vi "Init_Instr.vi"(8 "error in (no error)":errorcluster caption="entrée d'erreur (pas d'erreur)", 11 "Class Instrument Multimeter en entrée":refnum<class "Class Instrument Spectrum_Analyser.lvclass">) -> (0 "error out":errorcluster caption="sortie d'erreur", 3 "Class Instrument Multimeter en sortie":refnum<class "Class Instrument Spectrum_Analyser.lvclass">)   [LabVIEW 2020, in "Library Instrument & Equipement.lvlib" / "Library Instruments.lvlib" / "Class Instrument Spectrum_Analyser.lvclass"]
uses:
  Class Instrument Spectrum_Analyser.lvclass
  Class Instrument Spectrum_Analyser.lvclass/Class Instrument Spectrum_Analyser.ctl
  Instrument (Default)/Class Instrument (Default).lvclass
  Spectrum Analyser/Class Spectrum Analyser (Default)/Class Spectrum Analyser (Default).lvclass
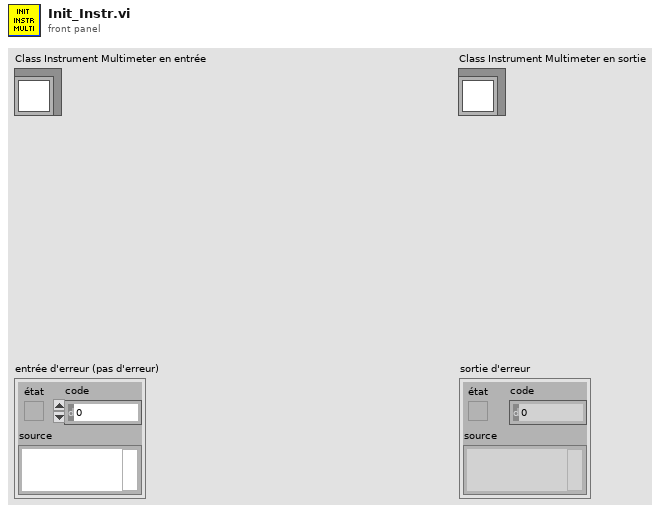
[diagram p1: front panel]
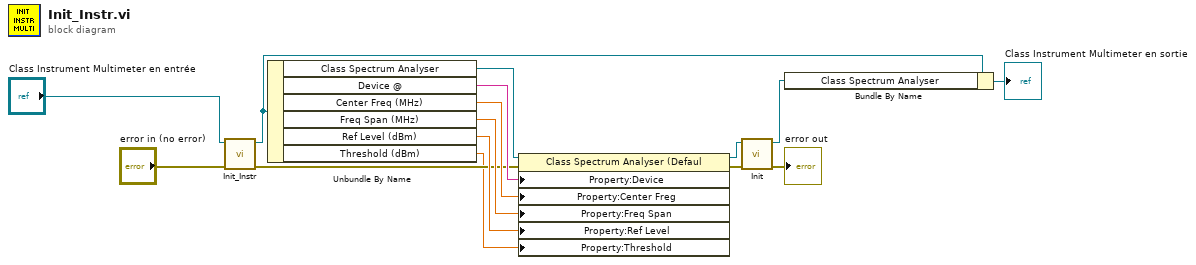
[diagram p0: block diagram]
diagram:
  n1 = call-parent "Init_Instr.vi"("error in (no error)"="error in (no error)", "Class Instrument (Default) en entrée"="Class Instrument Multimeter en entrée") -> ("error out"=w8:errorcluster, "Class Instrument (Default) en sortie"=w6:refnum<class "Class Instrument Spectrum_Analyser.lvclass">)  [unwired: 8 in]
  n2 = Unbundle By Name(w6) -> ("Class Spectrum Analyser"=w13:refnum<class "Class Spectrum Analyser (Default).lvclass">, "Device @"=w12:string, "Center Freq (MHz)"=w11:dbl, "Freq Span (MHz)"=w10:dbl, "Ref Level (dBm)"=w9:dbl, "Threshold (dBm)"=w1:dbl)
  n3 = property class="Class Spectrum Analyser (Defaul"(reference=w13, error in=w8, "Property:Device"=w12, "Property:Center Freg"=w11, "Property:Freq Span"=w10, "Property:Ref Level"=w9, "Property:Threshold"=w1) -> (reference out=w2:refnum<class "Class Spectrum Analyser (Default).lvclass">, error out=w5:errorcluster)
  n4 = call-dynamic "Init.vi"("error in (no error)"=w5, "Class Spectrum Analyser (Default) en entrée"=w2) -> ("error out"=→"error out":errorcluster, "Class Spectrum Analyser (Default) en sortie"=w3:refnum<class "Class Spectrum Analyser (Default).lvclass">)  [unwired: 8 in]
  n5 = Bundle By Name(cluster=w6, "Class Spectrum Analyser"=w3) -> (→"Class Instrument Multimeter en sortie":refnum<class "Class Instrument Spectrum_Analyser.lvclass">)
